vi "Update Lines.vi"(0 "Display State In":T1={"logTable"=refnum, "max items"=500, "displaydata"=[], "data"=[], "Auto Scroll"=TRUE, "current item"=500, "col headers"=[], "Add to Top"=TRUE, "Auto resize"=TRUE, "col size"=[], "filters"=[], "color cells"=[]}, 5 "Lines":string[][](array[string]), 7 "column":string, 9 "Container State":T3, 11 "error in (no error)":errorcluster) -> (4 "Display State Out":T1={"logTable"=refnum, "max items"=500, "displaydata"=[], "data"=[], "Auto Scroll"=TRUE, "current item"=500, "col headers"=[], "Add to Top"=TRUE, "Auto resize"=TRUE, "col size"=[], "filters"=[], "color cells"=[]}, 15 "error out":errorcluster)   [LabVIEW 2013, in "UI-DisplayTable(dev).xctl"]
uses:
  UI-DisplayTable(dev).xctl
  <vilib>/_xctls/Container State.ctl
  State.ctl
  Support/DEF-Filter.ctl
  <vilib>/_xctls/XControlSupport.lvlib
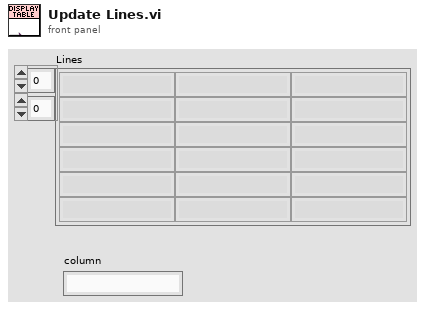
[diagram p1: front panel]
types:
  T1 = typedef "UI-DisplayTable(dev).xctl/State.ctl" = cluster{"logTable":refnum<vi>, "max items":i32, "displaydata":string[][], "data":string[][], "Auto Scroll":bool, "current item":i32, "col headers":string[], "Add to Top":bool, "Auto resize":bool, "col size":i32[], "filters":T2[], "color cells":cluster{"color cell":cluster{"Column":string, "Value":string, "Highlight Column":string}, "Color Box":u32}[]}
  T2 = typedef "UI-DisplayTable(dev).xctl/DEF-Filter.ctl" = cluster{"column":string, "value":string[]}
  T3 = typedef "XControlSupport.lvlib/Container State.ctl" = cluster{"Indicator?":bool, "Run Mode?":bool, " Refnum":refnum<vi>}
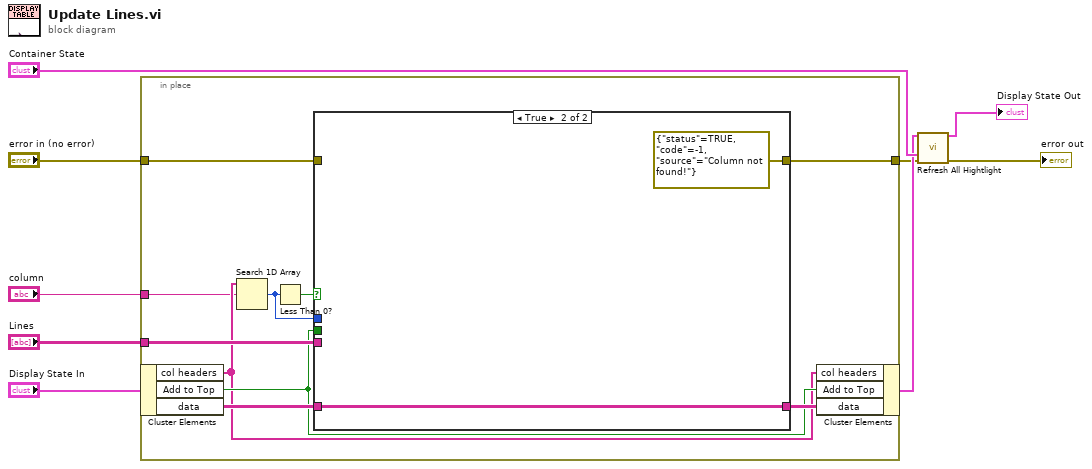
[diagram p0: block diagram]
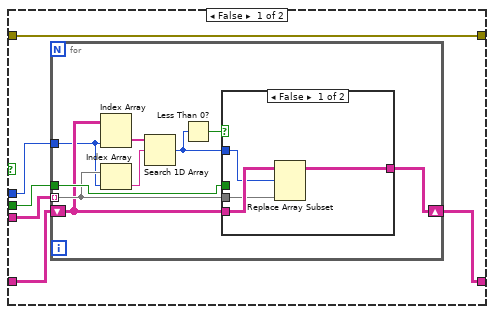
[diagram p2: hidden frame]
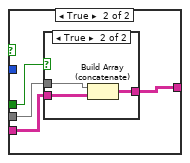
[diagram p3: hidden frame]
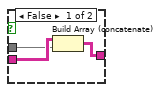
[diagram p4: hidden frame]
diagram:
  n1 = in-place {
    in-place-border: "Lines" -> [w18]
    in-place-border: "column" -> [w14]
    in-place-border: [w13] -> w2
    in-place-border: "error in (no error)" -> [w12]
    n2 = in-place-cluster #1("Display State In") -> ("col headers"=w15:string[], "Add to Top"=w16:bool, "data"=w19:string[][])
    n3 = Search 1D Array(1D array=w15, element=w14) -> (index of element=w10:i32)  [unwired: 1 in]
    n4 = Less Than 0?(x=w10) -> (x < 0?=w11:bool)
    n5 = case shown="True" w11 {
      tunnel: w19 -> [w21 w49]
      tunnel: w18 -> [w22 _]
      tunnel: [w25 w49] -> w17
      tunnel: w16 -> [w24 _]
      tunnel: [w23 errorcluster {"status"=TRUE, "code"=-1, "source"="Column not found!"} ("error in (no error)")] -> w13
      tunnel: w12 -> [w23 _]
      tunnel: w10 -> [w20 _]
      frame False {
        n6 = for {
          tunnel: w24 -> [w33]
          tunnel: w22 -> [w32] mode=indexing
          tunnel: w20 -> [w30]
          shift-right: [w34] -> w25
          shift-left: w21 -> [w31]
          n7 = Index Array(array=w31, index (col)=w30) -> (element=w29:string[])  [unwired: 1 in]
          n8 = Index Array(array=w32, index=w30) -> (element=w28:string)
          n9 = Search 1D Array(1D array=w29, element=w28) -> (index of element=w26:i32)  [unwired: 1 in]
          n10 = Less Than 0?(x=w26) -> (x < 0?=w27:bool)
          n11 = case shown="False" w27 {
            tunnel: [w36 w42] -> w34
            tunnel: w33 -> [_ w41]
            tunnel: w32 -> [w37 w40]
            tunnel: w31 -> [w38 w39]
            tunnel: w26 -> [w35 _]
            frame False {
              n12 = Replace Array Subset(array=w38, new element=w37, index (row)=w35) -> (w36:string[][])  [unwired: 1 in]
            }
            frame True {
              n13 = case shown="True" w41 {
                tunnel: w39 -> [w45 w48]
                tunnel: w40 -> [w44 w46]
                tunnel: [w43 w47] -> w42
                frame False {
                  n14 = Build Array (concatenate)(w45, w44) -> (w43:string[][])
                }
                frame True {
                  n15 = Build Array (concatenate)(w46, w48) -> (w47:string[][])
                }
              }
            }
          }
        }
      }
      frame True {
      }
    }
    n16 = in-place-cluster #1("col headers"=w15, "Add to Top"=w16, "data"=w17) -> (w4:T1)
  }
  n17 = call "Refresh All Hightlight.vi"("Display State In"=w4, "Container State"="Container State", "error in (no error)"=w2) -> ("Display State Out"=→"Display State Out":T1, "error out"=→"error out":errorcluster)  [unwired: 11 in]
